vi "Get Car Wash Started Event.vi"(8 "error in (no error)":errorcluster, 11 "Car Wash Started in":refnum<class "Car Wash Started.lvclass">) -> (0 "error out":errorcluster, 1 "Name":string, 3 "Wash Options":string[](array[string]))   [LabVIEW 2016, in "CLD Exam - Car Wash.lvlib" / "Car Wash Started.lvclass"]
uses:
  Car Wash Started.lvclass
  D:/Repos/Stream/software/Mediator/Classes/Message Interface/Message Interface.lvclass
  Car Wash Started.lvclass/Car Wash Started.ctl
  Mediator/Classes/Message Interface/Message Interface.lvclass
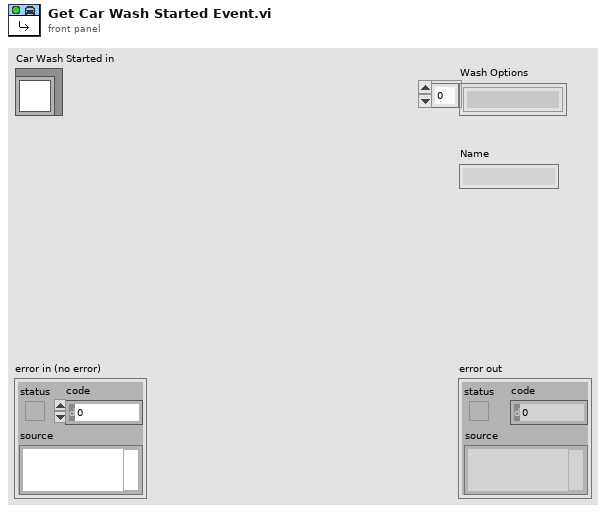
[diagram p1: front panel]
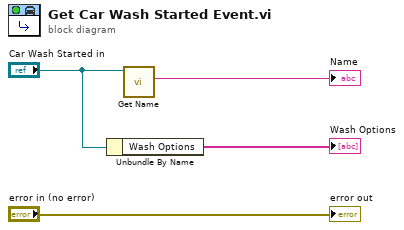
[diagram p0: block diagram]
diagram:
  n1 = Unbundle By Name("Car Wash Started in") -> ("Wash Options"=→"Wash Options":string[])
  n2 = call "Get Name.vi"("Message Interface in"="Car Wash Started in") -> ("Name"=→"Name":string)  [unwired: 8 in, 2 out]
  "error out" <- "error in (no error)"
